vi "Add Subpanel VI.vi"(8 "error in (no error)":errorcluster, 10 "subpanel VI":T1, 11 "VI Panel Layout in":refnum<class "VI Panel Layout.lvclass">) -> (0 "error out":errorcluster, 3 "VI Panel Layout out":refnum<class "VI Panel Layout.lvclass">)   [LabVIEW 2010, in "NI_SE_Front Panel Layout.lvlib" / "VI Panel Layout.lvclass"]
uses:
  VI Panel Layout.lvclass
  Subpanel VI Pair.ctl
  VI Panel Layout.lvclass/VI Panel Layout.ctl
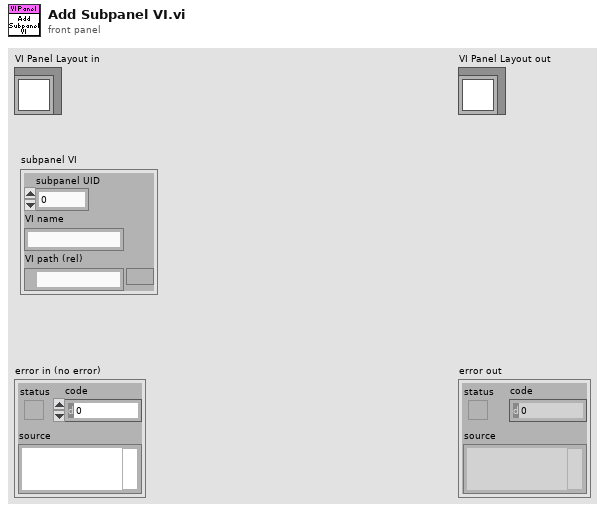
[diagram p1: front panel]
types:
  T1 = typedef "NI_SE_Front Panel Layout.lvlib/VI Panel Layout.lvclass/Subpanel VI Pair.ctl" = cluster{"subpanel UID":i32, "VI name":string, "VI path (rel)":path}
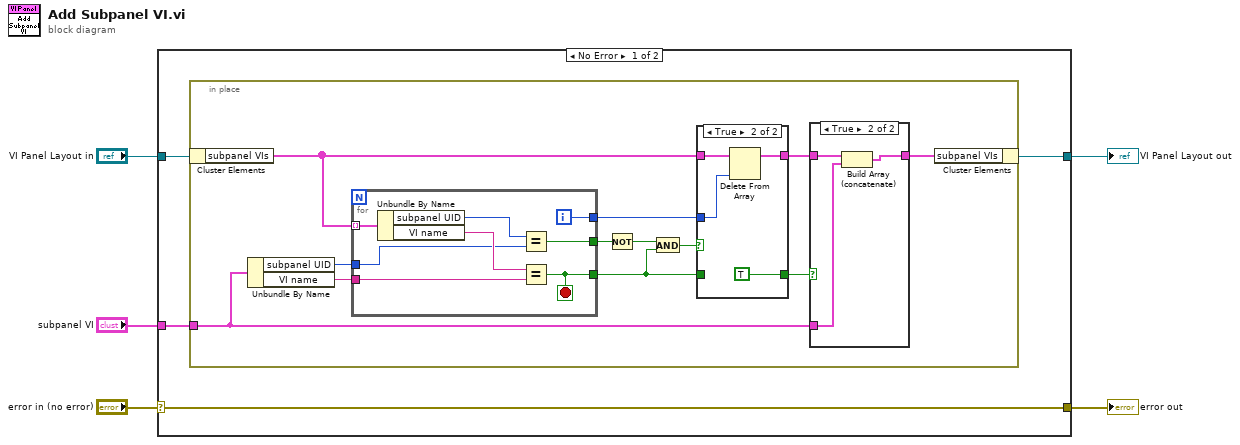
[diagram p0: block diagram]
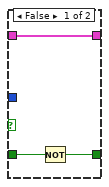
[diagram p2: hidden frame]
diagram:
  n1 = case shown="No Error" "error in (no error)" {
    selector: "error in (no error)" -> [w9 w42]
    tunnel: [w9 w42] -> w4
    tunnel: [w7 w41] -> w2
    tunnel: "VI Panel Layout in" -> [w8 w41]
    tunnel: "subpanel VI" -> [w6 _]
    frame No Error {
      n2 = in-place {
        in-place-border: w6 -> [w10]
        n3 = in-place-cluster #1(w8) -> ("subpanel VIs"=w17:T1[])
        n4 = Unbundle By Name(w10) -> ("subpanel UID"=w12:i32, "VI name"=w11:string)
        n5 = for {
          tunnel: w17 -> [w40] mode=indexing
          tunnel: w11 -> [w39]
          tunnel: w12 -> [w35]
          tunnel: [w37] -> w13
          tunnel: [w34] -> w20
          tunnel: [w33] -> w18
          i -> [w33]
          stop <- w37 stop-if-true
          n6 = Unbundle By Name(w40) -> ("subpanel UID"=w36:i32, "VI name"=w38:string)
          n7 = Equal?(x=w36, y=w35) -> (x = y?=w34:bool)
          n8 = Equal?(x=w38, y=w39) -> (x = y?=w37:bool)
        }
        n9 = Not(x=w20) -> (.not. x?=w16:bool)
        n10 = And(x=w16, y=w13) -> (x .and. y?=w19:bool)
        n11 = case shown="True" w19 {
          tunnel: w18 -> [_ w27]
          tunnel: w17 -> [w24 w28]
          tunnel: [w24 w26] -> w15
          tunnel: [w23 TRUE] -> w14
          tunnel: w13 -> [w22 _]
          frame False {
            n12 = Not(x=w22) -> (.not. x?=w23:bool)
          }
          frame True {
            n13 = Delete From Array(array=w28, index=w27) -> (array with subset deleted=w26:T1[])  [unwired: 1 in, 1 out]
          }
        }
        n14 = case shown="True" w14 {
          tunnel: w15 -> [w29 w32]
          tunnel: w10 -> [_ w31]
          tunnel: [w29 w30] -> w21
          frame False {
          }
          frame True {
            n15 = Build Array (concatenate)(w32, w31) -> (w30:T1[])
          }
        }
        n16 = in-place-cluster #1("subpanel VIs"=w21) -> (w7:refnum<class "VI Panel Layout.lvclass">)
      }
    }
    frame Error {
    }
  }
  "error out" <- w4
  "VI Panel Layout out" <- w2
